vi "addSpacing.vi"(8 "Error In":errorcluster, 10 "size":i32, 11 "QBoxLayout In":refnum<class "QBoxLayout.lvclass">) -> (0 "Error Out":errorcluster, 3 "QBoxLayout Out":refnum<class "QBoxLayout.lvclass">)   [LabVIEW 2014, in "QBoxLayout.lvclass"]
doc: "LabVIEW-specific documentation is not yet available. See <b>http://doc.qt.io/qt-5/QBoxLayout.html#addSpacing</b>"
uses:
  QBoxLayout.lvclass
  LQ Core/LQIdentity/LQIdentity.lvclass/LQIdentity.ctl
  LQ Core/LQ Core.lvlib
  LQ Core/LQIdentity/LQIdentity.lvclass
panel:
  # "Copyright (c) 2016 Sze Howe Koh\n\nThis Source Code Form is subject to the terms of the Mozilla Public\nLicense, v. 2.0. If a copy of the MPL was not distributed with this\nfile, You can obtain one at http://mozilla.org/MPL/2.0/."
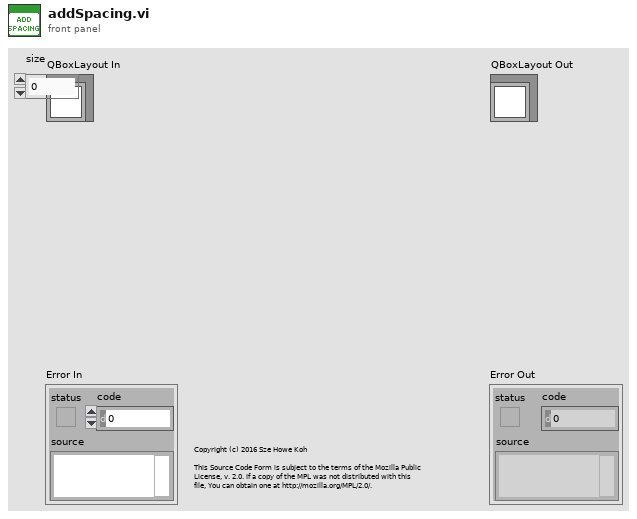
[diagram p1: front panel]
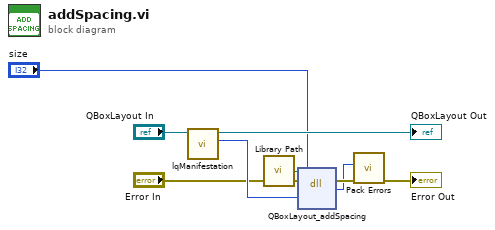
[diagram p0: block diagram]
diagram:
  n1 = call "lqManifestation.vi"("LQIdentity in"="QBoxLayout In") -> ("Manifestation"=w6:u64, "LQIdentity out"=→"QBoxLayout Out":refnum<class "QBoxLayout.lvclass">)  [unwired: 9 in]
  n2 = call "Library Path.vi"() -> ("Library Path"=w7:path)
  n3 = dll-call lib="?" fn="QBoxLayout_addSpacing"(path in=w7, error in="Error In", "_instance"=w6, "size"="size") -> (error out=w4:errorcluster, w2:i32)  [unwired: 3 in, 1 out]
  n4 = call "Pack Errors.vi"("Error In"=w4, "Error Code"=w2) -> ("Error Out"=→"Error Out":errorcluster)  [unwired: 9 in]
